vi "Stop Core.vi"(10 "final error code":i32, 11 "RootModel in":refnum<class "RootModel.lvclass">) -> (3 "RootModel out":refnum<class "RootModel.lvclass">)   [LabVIEW 2020, in "RootModel.lvlib" / "RootModel.lvclass"]
doc: "(<B>Filename</B>: Actor Framework.lvlib:Actor.lvclass:Stop Core.vi)\n\nDefines what the actor does before it stops. Use the <B>final error code</B> input to determine whether the actor shut down in response to an error.\n\nBy default, this method does nothing. A descendant class may override it to define behavior, such as shutting down any processes the actor initiated in its override of the Actor Core method."
uses:
  RootModel.lvclass
  RootModel.lvclass/RootModel.ctl
  IModel/IModel/IModel.lvclass
  IObserver/IObserver/IObserver.lvclass
  C:/Git/mva-core/Source/IModel/IModel/IModel.lvclass
  C:/Git/mva-core/Source/IObserver/IObserver/IObserver.lvclass
  C:/Program Files (x86)/National Instruments/LabVIEW 2020/vi.lib/ActorFramework/Actor/Actor.lvclass
  C:/Git/mva-core/Source/RootModel/RootModel/RootModel.lvclass
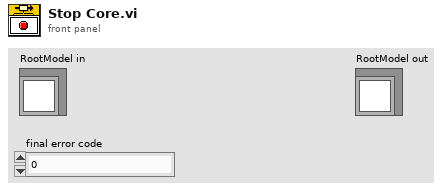
[diagram p1: front panel]
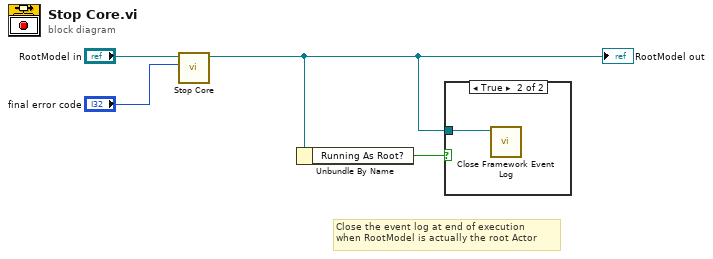
[diagram p0: block diagram]
diagram:
  # "Close the event log at end of execution\nwhen RootModel is actually the root Actor"
  n1 = call-parent "Stop Core.vi"("final error code"="final error code", "IObserver in"="RootModel in") -> ("IObserver out"=w2:refnum<class "RootModel.lvclass">)  [unwired: 9 in]
  "RootModel out" <- w2
  n2 = Unbundle By Name(w2) -> ("Running As Root?"=w1:bool)
  n3 = case shown="True" w1 {
    tunnel: w2 -> [_ w5]
    frame False {
    }
    frame True {
      n4 = call "Close Framework Event Log.vi"("IObserver in"=w5) -> ()  [unwired: 11 in]
    }
  }
